vi "checkResponsiveRobot.vi"() -> ()   [LabVIEW 2018]
uses:
  Intel/Functions Enum.ctl
  Intel/AttackerStates.ctl
  Path Planning/RRT/PathDest.ctl
  Path Planning/RRT/PathDests.ctl
  Core/AI Robot.ctl
  Core/AI Ball.ctl
  Core/Field Size.ctl
  Intel/Command Enum.ctl
  Core/AI Judge.ctl
  Util/Events/Events.ctl
  Core/AI Input.ctl
panel:
  out "Robots Status":cluster{"id":u32, bool}[](array[cluster])
  in  "IA State in":T1
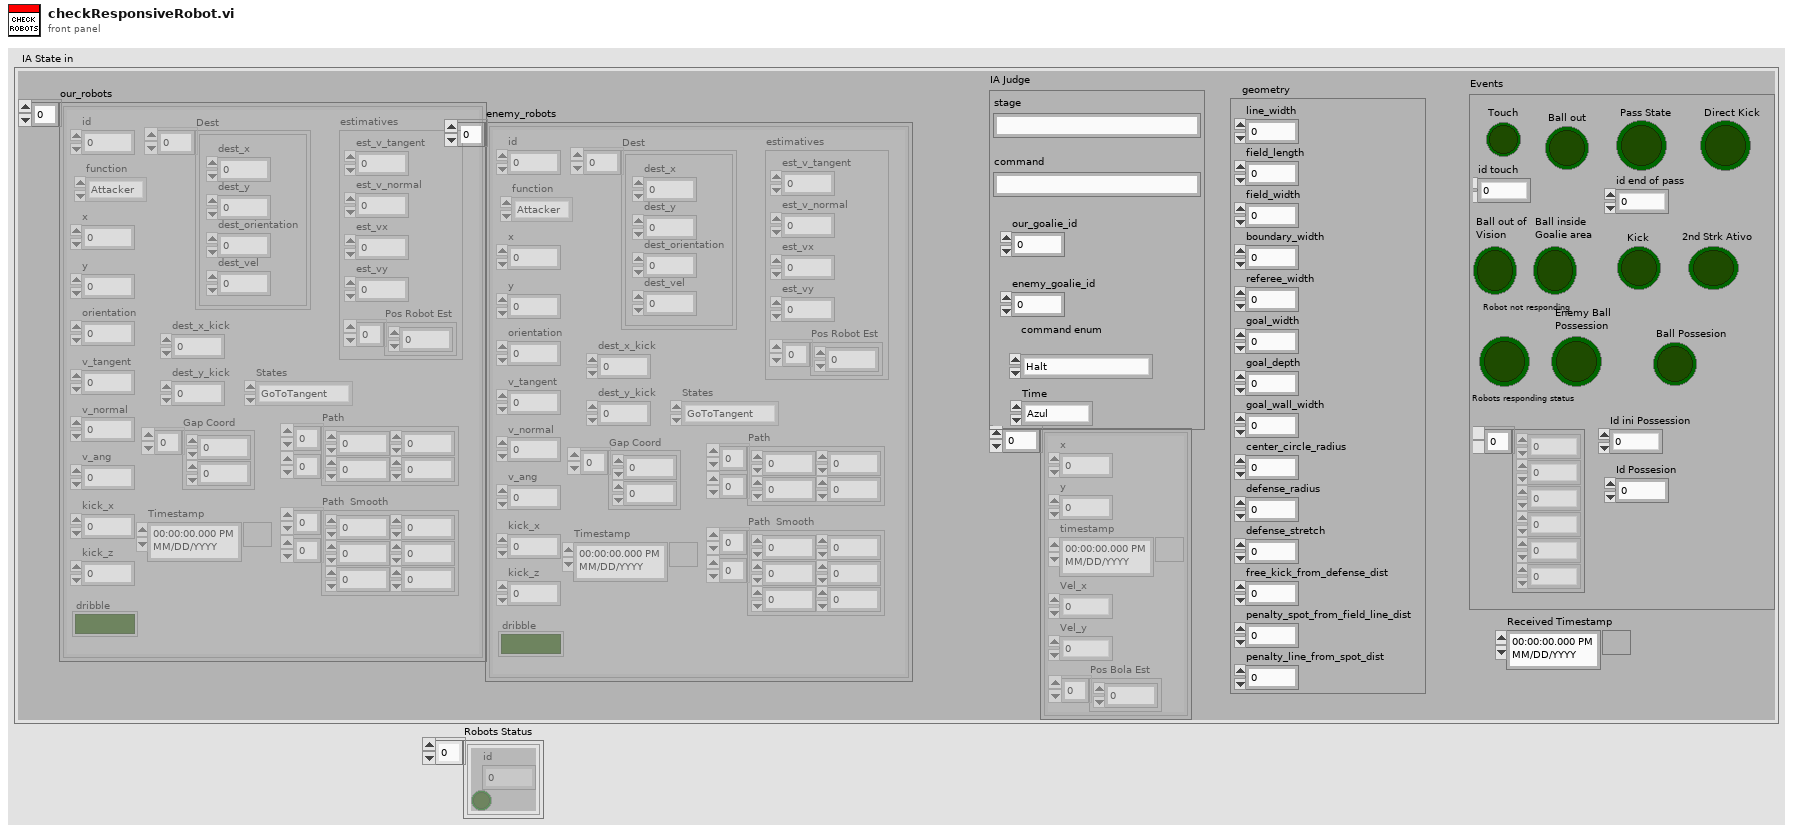
[diagram p1: front panel]
types:
  T1 = typedef "AI Input.ctl" = cluster{"our_robots":T2[], "enemy_robots":T2[], "balls":T7[], "geometry":T8, "IA Judge":T9, "Received Timestamp":timestamp, "Events":T11}
  T2 = typedef "AI Robot.ctl" = cluster{"id":u32, "function":T3, "x":dbl, "y":dbl, "orientation":dbl, "v_tangent":dbl, "v_normal":dbl, "v_ang":dbl, "kick_x":dbl, "kick_z":dbl, "dribble":bool, "Timestamp":timestamp, "estimatives":cluster{"est_v_tangent":dbl, "est_v_normal":dbl, "est_vx":dbl, "est_vy":dbl, "Pos Robot Est":dbl[]}, "dest_x_kick":dbl, "dest_y_kick":dbl, "Gap Coord":dbl[], "States":T4, "Path ":dbl[][], "Path  Smooth":dbl[][], "Dest":T5}
  T3 = typedef "Functions Enum.ctl" = enum16{"2nd Striker", "Attacker", "Goalie", "Defender", "Striker", "Goto 0", "Dummy", "Kicker", "ZigZag 0", "ZigZag 1", "ZigZag 2", "ZigZag 3", "ZigZag 4", "ZigZag 5", "ZigZag 6", "ZigZag 7", "ZigZag 8", ""}
  T4 = typedef "AttackerStates.ctl" = enum16{"Pass", "GoToTangent", "BallGetting", "GoToKick", ""}
  T5 = typedef "PathDests.ctl" = T6[]
  T6 = typedef "PathDest.ctl" = cluster{"dest_x":dbl, "dest_y":dbl, "dest_orientation":dbl, "dest_vel":dbl}
  T7 = typedef "AI Ball.ctl" = cluster{"x":dbl, "y":dbl, "timestamp":timestamp, "Vel_x":dbl, "Vel_y":dbl, "Pos Bola Est":dbl[]}
  T8 = typedef "Field Size.ctl" = cluster{"line_width":u32, "field_length":u32, "field_width":u32, "boundary_width":u32, "referee_width":u32, "goal_width":u32, "goal_depth":u32, "goal_wall_width":u32, "center_circle_radius":u32, "defense_radius":u32, "defense_stretch":u32, "free_kick_from_defense_dist":u32, "penalty_spot_from_field_line_dist":u32, "penalty_line_from_spot_dist":u32}
  T9 = typedef "AI Judge.ctl" = cluster{"stage":string, "command":string, "our_goalie_id":dbl, "enemy_goalie_id":dbl, "command enum":T10, "Time":enum16{"Azul", "Amarelo"}}
  T10 = typedef "Command Enum.ctl" = enum16{"Halt", "Stop", "Force Start", "PKA Normal Start", "Prepare Kickoff Ally", "PKE Normal Start", "Prepare Kickoff Enemy", "Prepare Penalty Ally", "PPA Normal Start", "Prepare Penalty Enemy", "PPE Normal Start", "Direct Free Enemy", "Direct Free Ally", "Indirect Free Enemy", "Indirect Free Ally", "Timeout Enemy", "Timeout Ally", "Goal Enemy", "Goal Ally", "Ball Placement Enemy", "Ball Placement Ally", "Normal Half Time", "Extra Time Break", "Extra Half Time", "None", "Post Game"}
  T11 = typedef "Events.ctl" = cluster{"Touch":bool, "Ball out":bool, "id touch":dbl, "Ball out of \nVision":bool, "Ball inside \nGoalie area":bool, "Robot not responding":bool, "Robots responding status":dbl[], "Enemy Ball \nPossession":bool, "Pass State":bool, "id end of pass":dbl, "Kick":bool, "Id ini Possession":dbl, "Ball Possesion":bool, "Id Possesion":dbl, "Direct Kick":bool, "2nd Strk Ativo":bool}
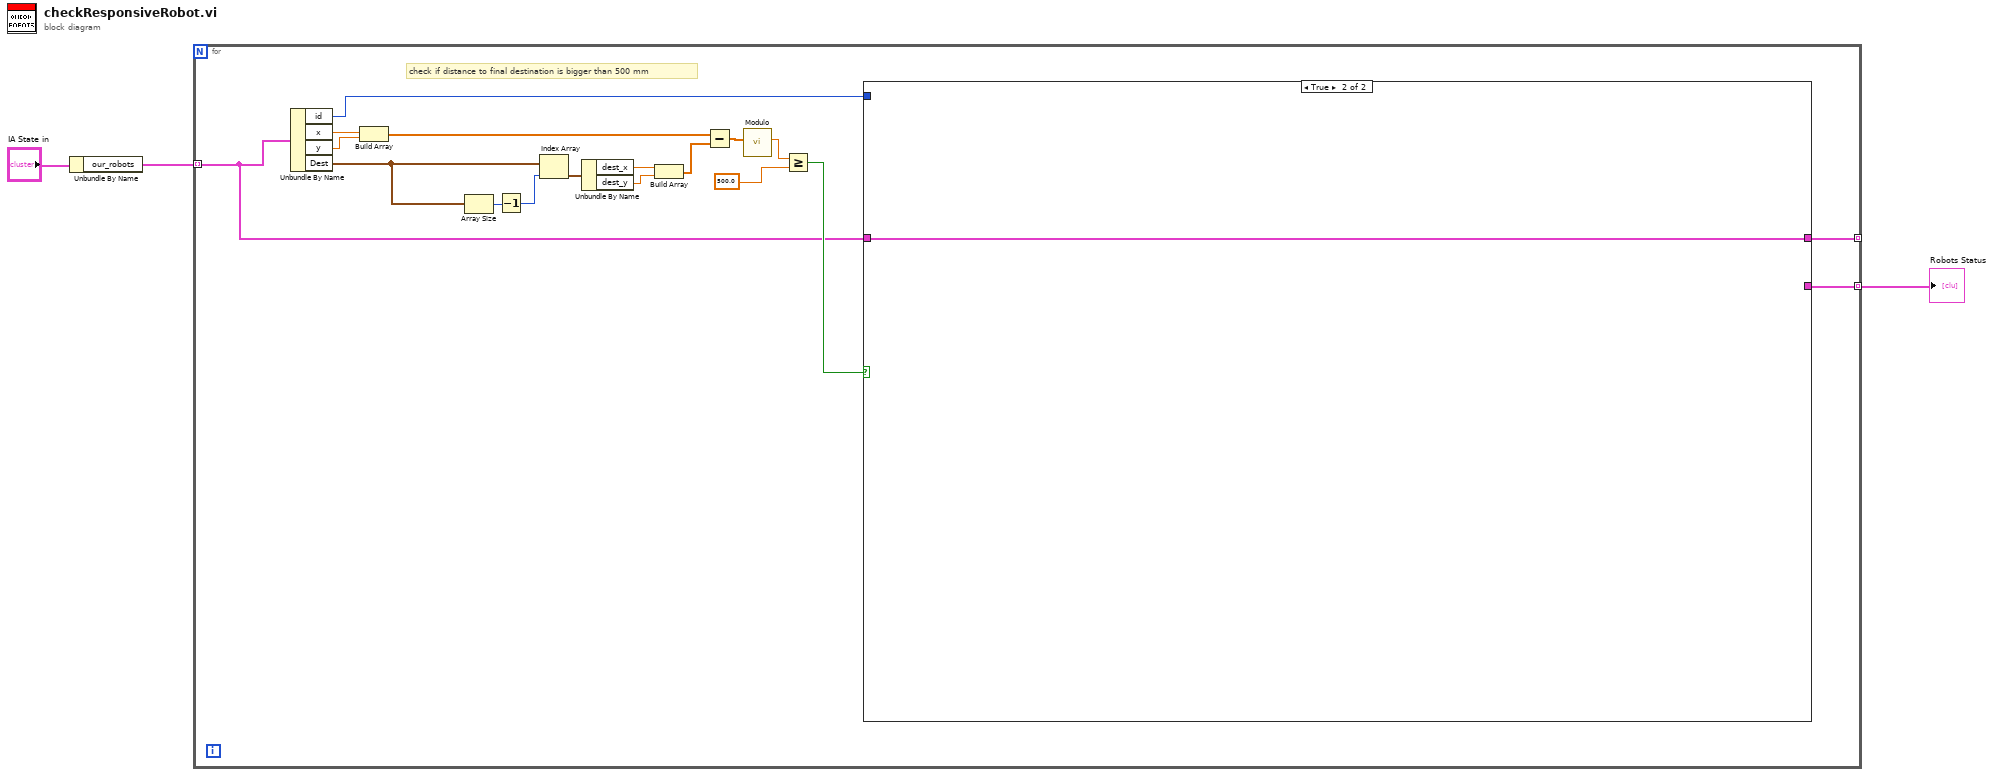
[diagram p0: block diagram]
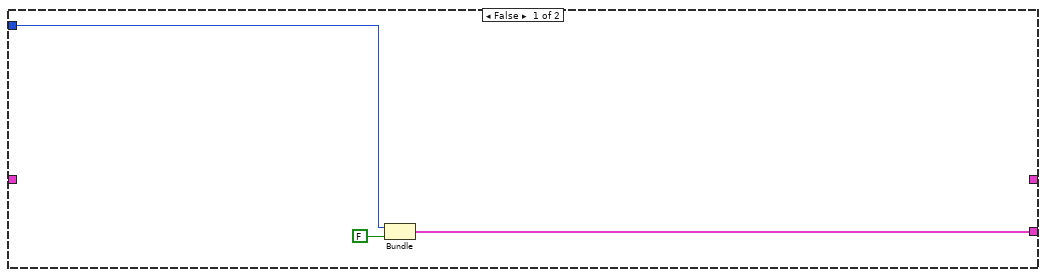
[diagram p2: hidden frame]
diagram:
  n1 = Unbundle By Name("IA State in") -> ("our_robots"=w2:T2[])
  n2 = for {
    tunnel: w2 -> [w4] mode=indexing
    tunnel: [w7] -> w1 mode=indexing
    tunnel: [w5] -> _ mode=indexing
    # "check if distance to final destination is bigger than 500 mm"
    n3 = Unbundle By Name(w4) -> ("id"=w8:u32, "x"=w18:dbl, "y"=w17:dbl, "Dest"=w21:T5)
    n4 = Build Array(w18, w17) -> (w13:dbl[])
    n5 = Array Size(array=w21) -> (size(s)=w20:i32)
    n6 = Decrement(x=w20) -> (x-1=w19:i32)
    n7 = Index Array(array=w21, index=w19) -> (element=w16:T6)
    n8 = Unbundle By Name(w16) -> ("dest_x"=w14:dbl, "dest_y"=w15:dbl)
    n9 = Build Array(w14, w15) -> (w6:dbl[])
    n10 = Subtract(x=w13, y=w6) -> (x-y=w12:dbl[])
    n11 = call "Modulo.vi"("2D vector"=w12) -> ("Modulo"=w11:dbl)  [unwired: 10 in]
    n12 = Greater Or Equal?(x=w11, y=500.0) -> (x >= y?=w9:bool)
    n13 = case shown="True" w9 {
      tunnel: w8 -> [w24 _]
      tunnel: [w22 _] -> w7
      tunnel: [_ w25] -> w5
      tunnel: w4 -> [_ w25]
      frame False {
        n14 = Bundle("id"=w24, FALSE) -> (w22:cluster{"id":u32, bool})  [unwired: 1 in]
      }
      frame True {
      }
    }
  }
  "Robots Status" <- w1
